vi "Byte To SCON.vi"(11 "Numeric":u8) -> (3 "SCON":T1)   [LabVIEW 2022 SP3, in "FHPP.lvclass"]
uses:
  FHPP.lvclass
  FHPP.lvclass/FHPP.ctl
  TypeDefs/SCON.ctl
  TypeDefs/Operating Mode.ctl
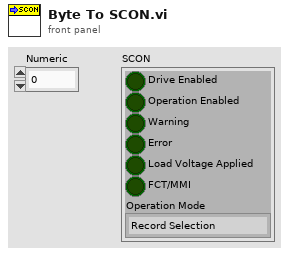
[diagram p1: front panel]
types:
  T1 = typedef "FHPP.lvclass/SCON.ctl" = cluster{"Drive Enabled":bool, "Operation Enabled":bool, "Warning":bool, "Error":bool, "Load Voltage Applied":bool, "FCT/MMI":bool, "Operation Mode":T2}
  T2 = typedef "FHPP.lvclass/Operating Mode.ctl" = enum16{"Record Selection", "Direct Mode", "Reserved 1", "Reserved 2"}
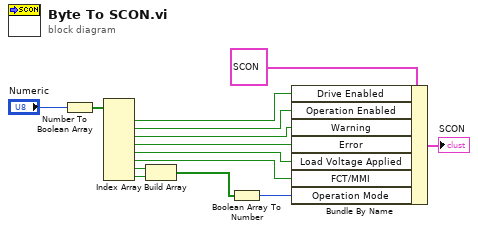
[diagram p0: block diagram]
diagram:
  n1 = Number To Boolean Array(number="Numeric") -> (Boolean array=w3:bool[])
  n2 = Index Array(array=w3) -> (element #1=w6:bool, element #2=w7:bool, element #3=w8:bool, element #4=w9:bool, element #5=w10:bool, element #6=w11:bool, element #7=w13:bool, element #8=w14:bool)  [unwired: 8 in]
  n3 = Build Array(w13, w14) -> (w1:bool[])
  n4 = Boolean Array To Number(Boolean array=w1) -> (number=w12:u32)
  n5 = Bundle By Name(cluster=T1 {"Drive Enabled"=FALSE, "Operation Enabled"=FALSE, "Warning"=FALSE, "Error"=FALSE, "Load Voltage Applied"=FALSE, "FCT/MMI"=FALSE, "Operation Mode"=enum."Record Selection"} ("SCON"), "Drive Enabled"=w6, "Operation Enabled"=w7, "Warning"=w8, "Error"=w9, "Load Voltage Applied"=w10, "FCT/MMI"=w11, "Operation Mode"=w12) -> (→"SCON":T1)
